vi "Delete Element.vi"(8 "error in (no error)":errorcluster, 10 "Delete Index":i32, 11 "Boolean_1D in":refnum<class "Boolean_1D.lvclass">) -> (0 "error out":errorcluster, 3 "Boolean_1D out":refnum<class "Boolean_1D.lvclass">)   [LabVIEW 2021, in "Boolean_1D.lvclass"]
uses:
  Boolean_1D.lvclass
  Boolean_1D.lvclass/Boolean_1D.ctl
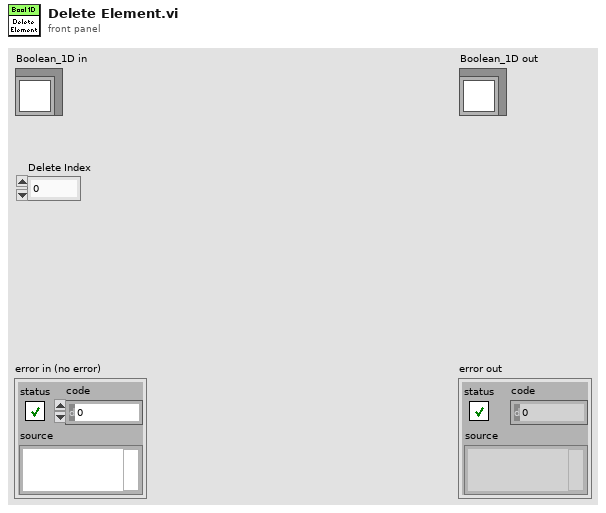
[diagram p1: front panel]
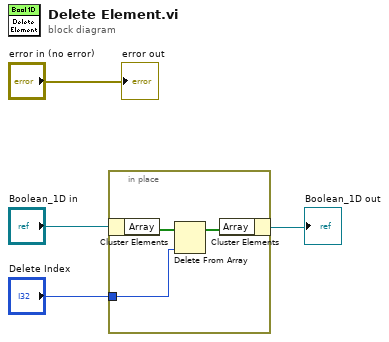
[diagram p0: block diagram]
diagram:
  n1 = in-place {
    in-place-border: "Delete Index" -> [w5]
    n2 = in-place-cluster #1("Boolean_1D in") -> ("Array"=w7:bool[])
    n3 = Delete From Array(array=w7, index=w5) -> (array with subset deleted=w6:bool[])  [unwired: 1 in, 1 out]
    n4 = in-place-cluster #1("Array"=w6) -> (→"Boolean_1D out":refnum<class "Boolean_1D.lvclass">)
  }
  "error out" <- "error in (no error)"
